vi "ROI entry screen-Delete ROIs.vi"(7 "No of lines I/p":i32, 9 "ROI Time (ns)":dbl, 10 "Deletion Idx":i32[](array[numeric]), 11 "ROI setup I/P":T1[](array[typedef]) {"Apparent Frame Size" format="%#_6f"; "Original FOV (um)" format="%#_6f"; "Pixels per miniscan" format="%#_6f"; "Dwell Time per pixel" format="%#_6f"; "Resolution" format="%#_6f"; "ROI group ID" format="%#_6f"; "Laser Power (%)" format="%#_6f"; "Zoom" format="%#_6f"; "Frame Size" format="%#_6f"; "Number of lines" format="%#_6f"; "Composite ID" format="%#_6f"; "Angle (deg)" format="%#_6f"; "ROI Time (ns)" format="%#_6f"; "ROI ID" format="%#_6f"; "Pixels in ROI" format="%#_6f"; "ROI index" format="%#_6f"; "Z stop" format="%#_6f"; "Y stop" format="%#_6f"; "X stop" format="%#_6f"; "Z start" format="%#_6f"; "X start" format="%#_6f"; "Y start" format="%#_6f"}) -> (1 "ROI Time (ns)o/p":dbl, 2 "No of ROIs":i32, 3 "ROI setup O/P":T1[](array[typedef]) {"Apparent Frame Size" format="%#_6f"; "Original FOV (um)" format="%#_6f"; "Pixels per miniscan" format="%#_6f"; "Dwell Time per pixel" format="%#_6f"; "Resolution" format="%#_6f"; "ROI group ID" format="%#_6f"; "Laser Power (%)" format="%#_6f"; "Zoom" format="%#_6f"; "Frame Size" format="%#_6f"; "Number of lines" format="%#_6f"; "Composite ID" format="%#_6f"; "Angle (deg)" format="%#_6f"; "ROI Time (ns)" format="%#_6f"; "ROI ID" format="%#_6f"; "Pixels in ROI" format="%#_6f"; "ROI index" format="%#_6f"; "Z stop" format="%#_6f"; "Y stop" format="%#_6f"; "X stop" format="%#_6f"; "Z start" format="%#_6f"; "X start" format="%#_6f"; "Y start" format="%#_6f"}, 5 "No of lines o/p":i32)   [LabVIEW 2020]
uses:
  Visualisation/Functional Imaging Viewer/Typedefs/ROI parameters data type.ctl
panel:
  out "Deleted ROIs":T1[](array[typedef]) {"Apparent Frame Size" format="%#_6f"; "Original FOV (um)" format="%#_6f"; "Pixels per miniscan" format="%#_6f"; "Dwell Time per pixel" format="%#_6f"; "Resolution" format="%#_6f"; "ROI group ID" format="%#_6f"; "Laser Power (%)" format="%#_6f"; "Zoom" format="%#_6f"; "Frame Size" format="%#_6f"; "Number of lines" format="%#_6f"; "Composite ID" format="%#_6f"; "Angle (deg)" format="%#_6f"; "ROI Time (ns)" format="%#_6f"; "ROI ID" format="%#_6f"; "Pixels in ROI" format="%#_6f"; "ROI index" format="%#_6f"; "Z stop" format="%#_6f"; "Y stop" format="%#_6f"; "X stop" format="%#_6f"; "Z start" format="%#_6f"; "X start" format="%#_6f"; "Y start" format="%#_6f"}
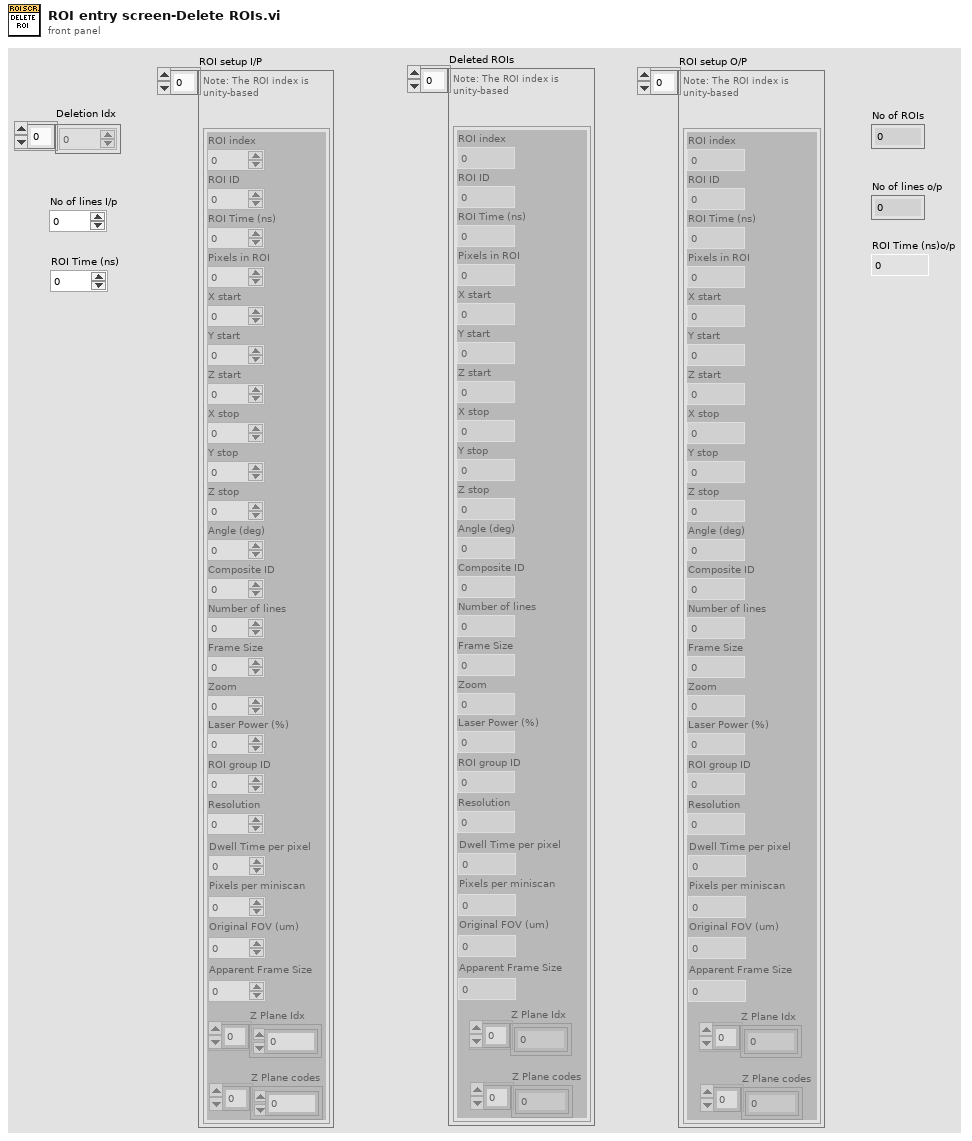
[diagram p1: front panel]
types:
  T1 = typedef "ROI parameters data type.ctl" = cluster{"ROI index":dbl, "ROI ID":dbl, "ROI Time (ns)":dbl, "Pixels in ROI":dbl, "X start":dbl, "Y start":dbl, "Z start":dbl, "X stop":dbl, "Y stop":dbl, "Z stop":dbl, "Angle (deg)":dbl, "Composite ID":dbl, "Number of lines":dbl, "Frame Size":dbl, "Zoom":dbl, "Laser Power (%)":dbl, "ROI group ID":dbl, "Resolution":dbl, "Dwell Time per pixel":dbl, "Pixels per miniscan":dbl, "Original FOV (um)":dbl, "Apparent Frame Size":dbl, "Z Plane Idx":i32[], "Z Plane codes":i32[]}
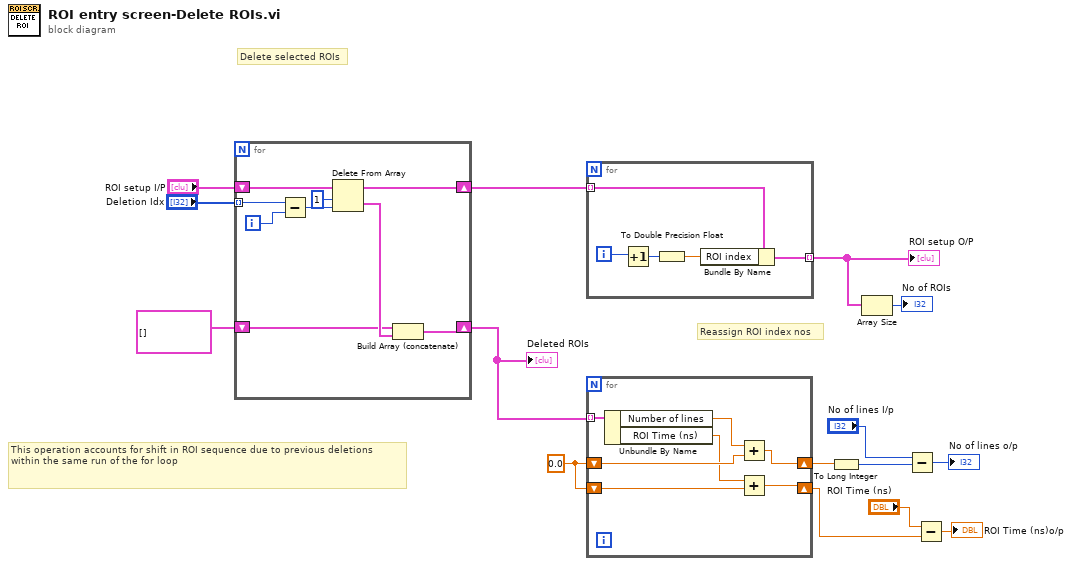
[diagram p0: block diagram]
diagram:
  w4 = 0.0
  # "Reassign ROI index nos"
  # "This operation accounts for shift in ROI sequence due to previous deletions\nwithin the same run of the for loop"
  # "Delete selected ROIs"
  n1 = for {
    shift-right: [w21] -> w12
    shift-left: "ROI setup I/P" -> [w22]
    tunnel: "Deletion Idx" -> [w20] mode=indexing
    shift-right: [w16] -> w9
    shift-left: T1[] [] -> [w17]
    i -> [w19]
    n2 = Subtract(x=w20, y=w19) -> (x-y=w24:i32)
    n3 = Delete From Array(array=w22, length=1, index=w24) -> (deleted portion=w18:T1[], array with subset deleted=w21:T1[])
    n4 = Build Array (concatenate)(w17, w18) -> (w16:T1[])
  }
  "Deleted ROIs" <- w9
  n5 = for {
    tunnel: w12 -> [w29] mode=indexing
    tunnel: [w25] -> w11 mode=indexing
    i -> [w28]
    n6 = Increment(x=w28) -> (x+1=w27:i32)
    n7 = To Double Precision Float(number=w27) -> (double precision float=w26:dbl)
    n8 = Bundle By Name(cluster=w29, "ROI index"=w26) -> (w25:T1)
  }
  "ROI setup O/P" <- w11
  n9 = for {
    tunnel: w9 -> [w36] mode=indexing
    shift-right: [w33] -> w8
    shift-left: w4 -> [w34]
    shift-right: [w30] -> w2
    shift-left: w4 -> [w31]
    n10 = Unbundle By Name(w36) -> ("Number of lines"=w35:dbl, "ROI Time (ns)"=w32:dbl)
    n11 = Add(x=w35, y=w34) -> (x+y=w33:dbl)
    n12 = Add(x=w32, y=w31) -> (x+y=w30:dbl)
  }
  n13 = To Long Integer(number=w8) -> (32bit integer=w6:i32)
  n14 = Array Size(array=w11) -> (size(s)=→"No of ROIs":i32)
  n15 = Subtract(x="No of lines I/p", y=w6) -> (x-y=→"No of lines o/p":i32)
  n16 = Subtract(x="ROI Time (ns)", y=w2) -> (x-y=→"ROI Time (ns)o/p":dbl)
